vi "process directories and files.vi"(8 "error in":errorcluster, 9 "include files in":variant, 10 "include directories":variant, 11 "Destination directory":path) -> (0 "error out":errorcluster)   [LabVIEW 2014]
uses:
  <vilib>/Utility/sysdir.llb/System Directory Type.ctl
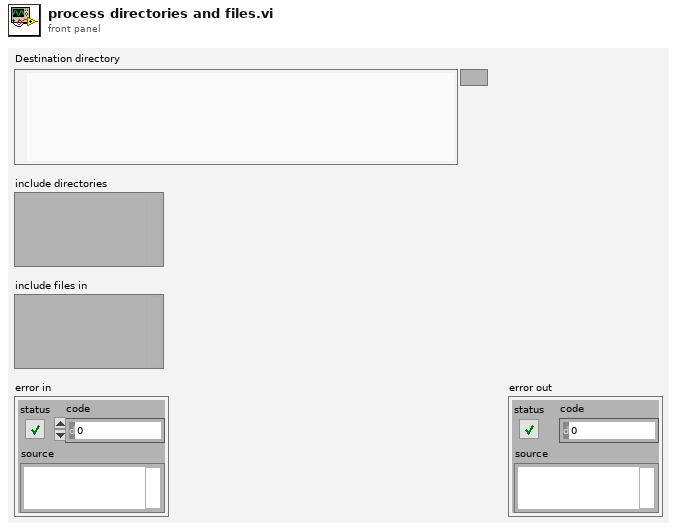
[diagram p1: front panel]
types:
  T1 = typedef "System Directory Type.ctl" = i32
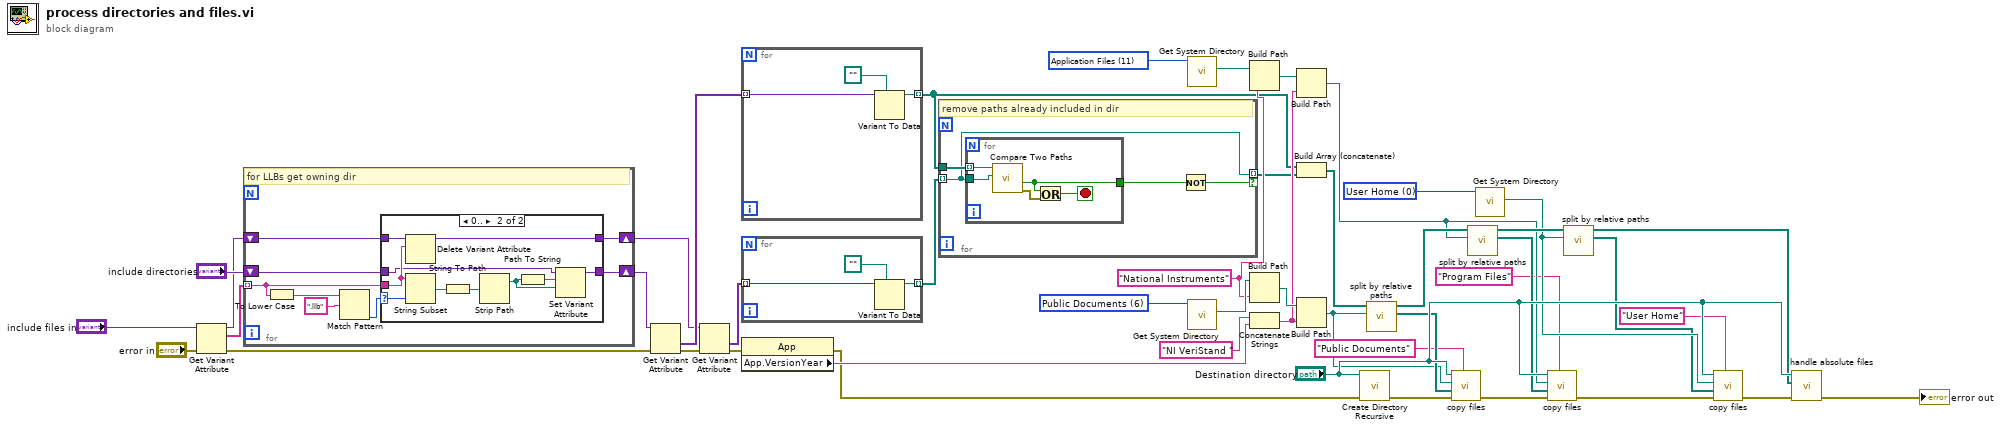
[diagram p0: block diagram]
diagram:
  w23 = T1 0 items=["User Home"=0, "User Desktop"=1, "User Documents"=2, "User Application Data"=3, "User Preferences"=4, "User Temporary"=5, "Public Documents"=6, "Public Application Data"=7, "Public Preferences"=8, "Public Cache"=13, "System Core Libraries"=9, "System Installed Libraries"=10, "Application Files"=11, "Boot Volume Root"=12] ("system directory type")
  w32 = T1 11 items=["User Home"=0, "User Desktop"=1, "User Documents"=2, "User Application Data"=3, "User Preferences"=4, "User Temporary"=5, "Public Documents"=6, "Public Application Data"=7, "Public Preferences"=8, "Public Cache"=13, "System Core Libraries"=9, "System Installed Libraries"=10, "Application Files"=11, "Boot Volume Root"=12] ("system directory type")
  w28 = "National Instruments"
  w37 = T1 6 items=["User Home"=0, "User Desktop"=1, "User Documents"=2, "User Application Data"=3, "User Preferences"=4, "User Temporary"=5, "Public Documents"=6, "Public Application Data"=7, "Public Preferences"=8, "Public Cache"=13, "System Core Libraries"=9, "System Installed Libraries"=10, "Application Files"=11, "Boot Volume Root"=12] ("system directory type")
  n1 = Get Variant Attribute(Variant="include files in", error in="error in") -> (duplicate Variant=w42:variant, names=w41:string[], error out=w21:errorcluster)  [unwired: 2 in, 1 out]
  n2 = for {
    shift-right: [w51] -> w43
    shift-left: "include directories" -> [w50]
    shift-right: [w48] -> w39
    shift-left: w42 -> [w49]
    tunnel: w41 -> [w47] mode=indexing
    # "for LLBs get owning dir"
    n3 = To Lower Case(string=w47) -> (all lower case string=w53:string)
    n4 = Match Pattern(string=w53, regular expression=".llb") -> (offset past match=w52:i32)  [unwired: 1 in, 3 out]
    n5 = case shown="0.." w52 {
      selector: w52 -> [_ w63]
      tunnel: [w56 w60] -> w51
      tunnel: w50 -> [w56 w59]
      tunnel: w49 -> [w55 w66]
      tunnel: [w55 w65] -> w48
      tunnel: w47 -> [_ w64]
      frame ..-1 {
      }
      frame 0.. {
        n6 = Delete Variant Attribute(6:w64, 7:w66) -> (3:w65:variant)  [unwired: 1 in, 2 out]
        n7 = String Subset(string=w64, length (rest)=w63) -> (substring=w62:string)  [unwired: 1 in]
        n8 = String To Path(string=w62) -> (path=w61:path)
        n9 = Strip Path(path=w61) -> (stripped path=w57:path)  [unwired: 1 out]
        n10 = Path To String(path=w57) -> (string=w58:string)
        n11 = Set Variant Attribute(Variant=w59, name=w58, value=w57) -> (Variant out=w60:variant)  [unwired: 1 in, 2 out]
      }
    }
  }
  n12 = Get Variant Attribute(Variant=w43, error in=w21) -> (values=w46:variant[], error out=w19:errorcluster)  [unwired: 2 in, 2 out]
  n13 = Get Variant Attribute(Variant=w39, error in=w19) -> (values=w40:variant[], error out=w18:errorcluster)  [unwired: 2 in, 2 out]
  n14 = for {
    tunnel: w46 -> [w69] mode=indexing
    tunnel: [w67] -> w27 mode=indexing
    n15 = Variant To Data(type=path "", Variant=w69) -> (data=w67:path)  [unwired: 1 in, 1 out]
  }
  n16 = for {
    tunnel: w40 -> [w72] mode=indexing
    tunnel: [w70] -> w38 mode=indexing
    n17 = Variant To Data(type=path "", Variant=w72) -> (data=w70:path)  [unwired: 1 in, 1 out]
  }
  n18 = property class="App"(error in=w18) -> (error out=w17:errorcluster, "App.VersionYear"=w34:string)  [unwired: 1 in, 1 out]
  n19 = for {
    tunnel: w38 -> [w75] mode=indexing
    tunnel: w27 -> [w76]
    tunnel: [w75] -> w26 mode=indexing if=w73
    # "remove paths already included in dir"
    n20 = for {
      tunnel: w76 -> [w81] mode=indexing
      tunnel: w75 -> [w80]
      tunnel: [w79] -> w74
      stop <- w78 stop-if-true
      n21 = call <vilib>:"Compare Two Paths.vi"("Path 2"=w80, "Path 1"=w81) -> ("error out"=w77:errorcluster, "Path 2 Relative to Path 1?"=w79:bool)  [unwired: 6 in, 2 out]
      n22 = Or(x=w79, y=w77) -> (x .or. y?=w78:bool)
    }
    n23 = Not(x=w74) -> (.not. x?=w73:bool)
  }
  n24 = call <vilib>:"Get System Directory.vi"("system directory type"=w32) -> ("system directory"=w31:path)  [unwired: 10 in]
  n25 = call <vilib>:"Get System Directory.vi"("system directory type"=w37) -> ("system directory"=w36:path)  [unwired: 10 in]
  n26 = Build Path(base path=w31, name or relative path=w28) -> (appended path=w30:path)
  n27 = Build Path(base path=w36, name or relative path=w28) -> (appended path=w35:path)
  n28 = Concatenate Strings("NI VeriStand ", w34) -> (w29:string)
  n29 = Build Path(base path=w30, name or relative path=w29) -> (appended path=w12:path)
  n30 = Build Array (concatenate)(w27, w26) -> (w25:path[])
  n31 = Build Path(base path=w35, name or relative path=w29) -> (appended path=w13:path)
  n32 = call <vilib>:"Create Directory Recursive.vi"("error in (no error)"=w17, "directory"="Destination directory") -> ("error out"=w15:errorcluster)  [unwired: 3 in, 2 out]
  n33 = call "split by relative paths.vi"("base path"=w13, "paths to search"=w25) -> ("relative"=w14:path[], "not relative"=w24:path[])  [unwired: 7 in, 1 out]
  n34 = call "copy files.vi"("relative"="Public Documents" ("name or relative path"), "error in"=w15, "files in base path"=w14, "base path"=w13, "destination path"="Destination directory") -> ("error out"=w9:errorcluster)  [unwired: 6 in]
  n35 = call "split by relative paths.vi"("base path"=w12, "paths to search"=w24) -> ("relative"=w11:path[], "not relative"=w22:path[])  [unwired: 7 in, 1 out]
  n36 = call <vilib>:"Get System Directory.vi"("system directory type"=w23) -> ("system directory"=w8:path)  [unwired: 10 in]
  n37 = call "copy files.vi"("relative"="Program Files" ("name or relative path"), "error in"=w9, "files in base path"=w11, "base path"=w12, "destination path"="Destination directory") -> ("error out"=w10:errorcluster)  [unwired: 6 in]
  n38 = call "split by relative paths.vi"("base path"=w8, "paths to search"=w22) -> ("relative"=w7:path[], "not relative"=w5:path[])  [unwired: 7 in, 1 out]
  n39 = call "copy files.vi"("relative"="User Home" ("name or relative path"), "error in"=w10, "files in base path"=w7, "base path"=w8, "destination path"="Destination directory") -> ("error out"=w6:errorcluster)  [unwired: 6 in]
  n40 = call "handle absolute files.vi"("error in"=w6, "absolute files"=w5, "destination directory"="Destination directory") -> ("error out"=→"error out":errorcluster)  [unwired: 8 in]
